vi "20T_Change_Switch_Heater_Status.vi"(8 "error in (no error)":errorcluster, 11 "Mercury Reference In":T1) -> (0 "error out":errorcluster)   [LabVIEW 2019]
uses:
  Equipment/Mercury iXX/Public/Controls/Mercury Reference.ctl
  Equipment/Mercury iXX/Public/Controls/Comms Transport Layer.ctl
  Equipment/Mercury iXX/Private/Controls/Query Dynamic Reference.ctl
  Equipment/Mercury iXX/Public/Libraries/Magnet/Open/Open Magnet Device.vi
  Equipment/Mercury iXX/Public/Libraries/Magnet/Signals/Read/Persistant Field (Read).vi
  Equipment/Mercury iXX/Public/Libraries/Magnet/Signals/Read/Field (Read).vi
  Equipment/Mercury iXX/Public/Libraries/Magnet/Signals/Read/Switch Heater Status (Read).vi
  Equipment/Mercury iXX/Mercury iXX.lvlib
  Equipment/Mercury iXX/Public/Libraries/Magnet.lvlib
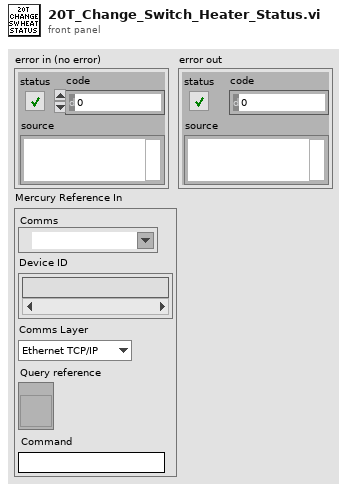
[diagram p1: front panel]
types:
  T1 = typedef "Mercury iXX.lvlib/Mercury Reference.ctl" = cluster{"Comms":refnum<visa-resource-name>, "Device ID":string[], "Comms Layer":T2, "Command":string, "Query reference":T3}
  T2 = typedef "Mercury iXX.lvlib/Comms Transport Layer.ctl" = enum16{"Ethernet TCP/IP", "USB", "ISOBus - RS-232", "GPIB"}
  T3 = typedef "Mercury iXX.lvlib/Query Dynamic Reference.ctl" = refnum<vi>
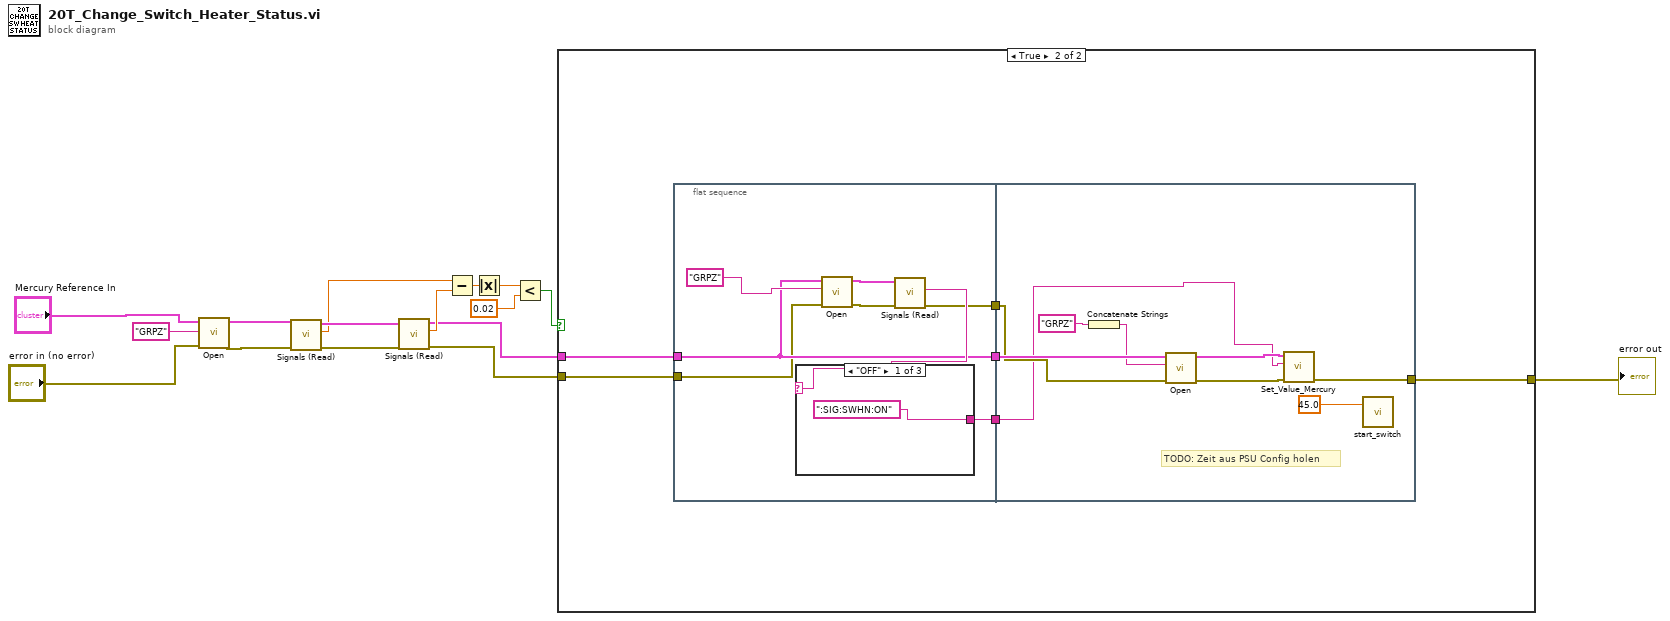
[diagram p0: block diagram]
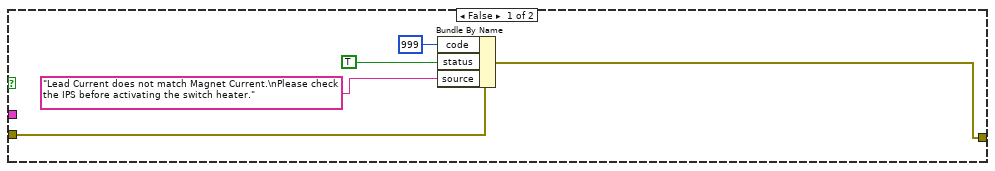
[diagram p2: hidden frame]
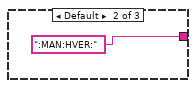
[diagram p3: hidden frame]
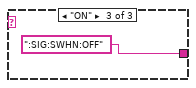
[diagram p4: hidden frame]
diagram:
  n1 = call-poly "Open.vi"("error in (no error)"="error in (no error)", "Device Identifier"="GRPZ", "Mercury Reference In"="Mercury Reference In") -> ("error out"=w14:errorcluster, "Mercury Reference Out"=w13:T1)  [unwired: 1 in, 6 out]
  n2 = call-poly "Signals (Read).vi"("error in"=w14, "Mercury Reference In"=w13) -> ("error out"=w10:errorcluster, "Persistant Field"=w8:dbl, "Mercury Reference Out"=w12:T1)  [unwired: 5 in, 2 out]
  n3 = call-poly "Signals (Read).vi"("error in"=w10, "Mercury Reference In"=w12) -> ("error out"=w9:errorcluster, "Field"=w7:dbl, "Mercury Reference Out"=w3:T1)  [unwired: 5 in, 2 out]
  n4 = Subtract(x=w8, y=w7) -> (x-y=w6:dbl)
  n5 = Absolute Value(x=w6) -> (abs(x)=w5:dbl)
  n6 = Less?(x=w5, y=0.02) -> (x < y?=w4:bool)
  n7 = case shown="True" w4 {
    tunnel: w3 -> [_ w24]
    tunnel: w9 -> [w20 w23]
    tunnel: [w19 w22] -> w1
    frame False {
      n8 = Bundle By Name(cluster=w20, "code"=999, "status"=TRUE, "source"="Lead Current does not match Magnet Current.\nPlease check the IPS before activating the switch heater.") -> (w19:errorcluster)
    }
    frame True {
      n9 = flat-sequence {
        tunnel: w24 -> [w31]
        tunnel: [w31] -> w27
        tunnel: w23 -> [w30]
        tunnel: [w29] -> w26
        tunnel: [w28] -> w25
        tunnel: w27 -> [w47]
        tunnel: w26 -> [w44]
        tunnel: w25 -> [w40]
        tunnel: [w39] -> w22
        frame #0 {
          n10 = call-poly "Open.vi"("error in (no error)"=w30, "Device Identifier"="GRPZ", "Mercury Reference In"=w31) -> ("error out"=w32:errorcluster, "Mercury Reference Out"=w33:T1)  [unwired: 1 in, 6 out]
          n11 = call-poly "Signals (Read).vi"("error in"=w32, "Mercury Reference In"=w33) -> ("error out"=w29:errorcluster, "Switch Heater Status"=w35:string)  [unwired: 6 in, 2 out]
          n12 = case shown="\"OFF\"" w35 {
            tunnel: [":SIG:SWHN:ON" ":MAN:HVER:" ":SIG:SWHN:OFF"] -> w28
            frame "OFF" {
            }
            frame Default {
            }
            frame "ON" {
            }
          }
        }
        frame #1 {
          # "TODO: Zeit aus PSU Config holen"
          n13 = Concatenate Strings("GRPZ" ("Device Identifier")) -> (w46:string)
          n14 = call-poly "Open.vi"("error in (no error)"=w44, "Device Identifier"=w46, "Mercury Reference In"=w47) -> ("error out"=w42:errorcluster, "Mercury Reference Out"=w41:T1)  [unwired: 1 in, 6 out]
          n15 = call "Set_Value_Mercury.vi"("error in"=w42, "Noun(s)"=w40, "Mercury Reference In"=w41) -> ("error out"=w39:errorcluster)  [unwired: 7 in, 1 out]
          n16 = call "start_switch.vi"("Switch heater time"=45.0) -> ()  [unwired: 2 in]
        }
      }
    }
  }
  "error out" <- w1
